vi "set_material_name.vi"(8 "error in (no error)":errorcluster, 9 "Material name":string, 10 "Material number":u8, 11 "VISA resource name":refnum<visa-resource-name>) -> (0 "error out":errorcluster, 3 "VISA resource name out":refnum<visa-resource-name>)   [LabVIEW 2018]
doc: "Update the name of an output."
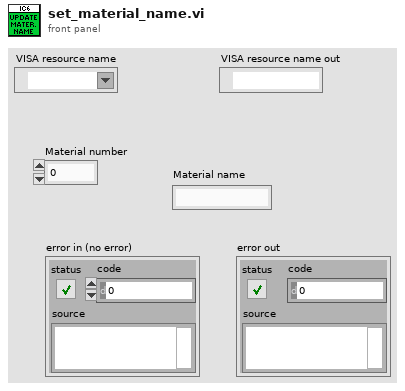
[diagram p1: front panel]
types:
  T1 = enum16{"Source", "General", "Input name", "Process name", "Logic", "Material", "Material name", "Output name", "Process", "Sensor", "Output type", "User message", "Layer", ""}
  T2 = enum16{"Hello", "Query", "Remote action", "Status", "Update"}
  T3 = cluster{"Material number":u8, "Material name":string}
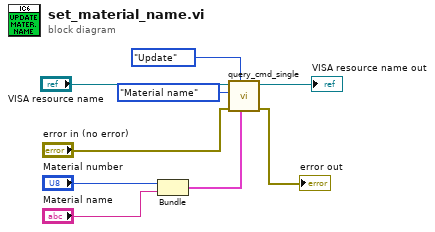
[diagram p0: block diagram]
diagram:
  n1 = Bundle("Material number"="Material number", "Material name"="Material name") -> (w1:T3)  [unwired: 1 in]
  n2 = call "query_cmd_single.vi"("Parameter"=w1, "Command group"=T2."Update", "error in (no error)"="error in (no error)", "Command subgroup"=T1."Material name", "VISA resource name"="VISA resource name") -> ("error out"=→"error out":errorcluster, "VISA resource name out"=→"VISA resource name out":refnum<visa-resource-name>)  [unwired: 2 in, 3 out]
